vi "UHR-Fleezers Control (host) - Lorentz v4.vi"() -> ()   [LabVIEW 2014] (continued)
        n2223 = Multiply(x="Base N trap periods", y="Period scale factor") -> ()  [unwired: 1 out]
        n2224 = local read "Cal sets to save"() -> (w3460:u32)
        n2225 = To Unsigned Quad Integer(1:w3456) -> (0:w3446:u64)
        n2226 = for "vector 0 to N -1" {
          N: w3432 -> [_]
          tunnel: [w3481] -> w3452 mode=indexing
          i -> [w3481]
        }
        n2227 = Multiply "Ticks/DMA"(x=w3459, y=w3464) -> (x*y=w3463:u32)
        n2228 = Multiply "Scaled osc period (s)"(x=w3446, y=2.5e-08) -> (x*y=w3458:dbl)
        "Trap OSC Period (s)" <- w3458
        n2229 = Reciprocal(x=w3458) -> (1/x=→"A cal freq (Hz)":dbl)
        n2230 = Multiply(x=w3452, y=6.283185307179586) -> (x*y=w3467:dbl[])
        n2231 = Quotient & Remainder(x=w3463, y=w3446) -> (x-y*floor(x/y)=w3439:u64, floor(x/y)=→"N osc / DMA":u64)
        "DMA remainder" <- w3439
        n2232 = Multiply "Total trap ticks"(x=w3460, y=w3463) -> (x*y=w3447:u32)
        n2233 = Divide(x=w3467, y=w3432) -> (x/y=w3468:dbl[])
        n2234 = Sine(x=w3468) -> (sin(x)=w3469:dbl[])
        n2235 = Quotient & Remainder(x=w3447, y=100) -> (x-y*floor(x/y)=w3442:u32, floor(x/y)=w3462:u32)
        "Total save/100 remainder" <- w3442
        n2236 = Multiply "Single period osc vector"(x=w3469, y="Trap osc amp (MHz)") -> (x*y=w3445:dbl[])
        n2237 = Quotient & Remainder(x=w3462, y=w3446) -> (x-y*floor(x/y)=w3441:u64, floor(x/y)=→"N osc/ (total save/100)":u64)
        "(total save/100) /osc period remainder" <- w3441
        n2238 = Quotient & Remainder(x=w3447, y=w3446) -> (x-y*floor(x/y)=w3440:u64)  [unwired: 1 out]
        "N trap osc periods per save remainder" <- w3440
        n2239 = call "IR AOM freq to word - vec.vi"("Frequency In (double vec, MHz)"=w3445) -> ("Frequency Word Out"=w3444:dbl[])
        n2240 = To Quad Integer(1:w3444) -> (0:w3443:i64[])
        n2241 = disable-structure shown="Disabled" {
          disable-tunnel: w3451 -> [w3473 _]
          disable-tunnel: w3443 -> [w3471 _]
          frame Disabled {
            n2242 = xnode "Read/Write Control"("FPGA VI Reference In"=w3473) -> ("FPGA VI Reference Out"=w3472:T50)  [unwired: 3 in, 1 out]
            n2243 = flat-sequence {
              tunnel: w3471 -> [w3476]
              tunnel: w3472 -> [w3475]
              frame #0 {
                n2244 = for "Write data to fpga memory" {
                  tunnel: w3475 -> [w3478]
                  tunnel: w3476 -> [_] mode=indexing
                  (unwired) TRUE ("Ready Write")
                  n2245 = xnode "Read/Write Control"("FPGA VI Reference In"=w3478) -> ("FPGA VI Reference Out"=w3477:T50)  [unwired: 4 in, 1 out]
                  n2246 = while {
                    tunnel: w3477 -> [w3479]
                    stop <- _ continue-if-true
                    n2247 = xnode "Read/Write Control"("FPGA VI Reference In"=w3479) -> ()  [unwired: 1 in, 3 out]
                  }
                }
                "Writing waveform to fpga memory" <- TRUE ("Writing waveform to fpga memory")
              }
              frame #1 {
                n2248 = local write "Writing waveform to fpga memory"(FALSE ("Writing waveform to fpga memory")) -> ()
              }
            }
          }
          frame Enabled {
          }
        }
        n2249 = Equal?(x=w3441, y=w3438) -> (x = y?=w3436:bool)
        n2250 = Equal?(x=w3442, y=w3438) -> (x = y?=w3437:bool)
        n2251 = Equal?(x=w3439, y=w3438) -> (x = y?=w3434:bool)
        n2252 = Equal?(x=w3440, y=w3438) -> (x = y?=w3435:bool)
        n2253 = Compound Arithmetic op=AND(w3437, w3436, w3435, w3434) -> (→"Good freq?":bool)
      }
      event "Osc trap cont.", "Osc traps", "T1 Osc Enable", "T2 Osc Enable": Value Change {
        n2254 = event-data() -> ()  [unwired: 7 out]
        n2255 = disable-structure shown="Disabled" {
          disable-tunnel: w3482 -> [w3485 _]
          frame Disabled {
            n2256 = xnode "Read/Write Control"("FPGA VI Reference In"=w3485, "Trap 1 osc enable"="T1 Osc Enable", "Trap 2 osc enable"="T2 Osc Enable") -> ()  [unwired: 1 in, 2 out]
          }
          frame Enabled {
          }
        }
      }
      event "Pressure Pump Voltage (+/-10V)": Value Change {
        n2257 = event-data() -> ()  [unwired: 7 out]
        n2258 = disable-structure shown="Disabled" {
          disable-tunnel: w3486 -> [w3490 _]
          frame Disabled {
            n2259 = Divide(x="Pressure Pump Voltage (+/-10V)", y=10.0) -> (x/y=w3487:dbl)
            n2260 = Multiply(x=w3487, y=32767.0) -> (x*y=w3488:dbl)
            n2261 = xnode "Read/Write Control"("FPGA VI Reference In"=w3490, "Pressure Pump"=w3488) -> ()  [unwired: 1 in, 2 out]
          }
          frame Enabled {
          }
        }
      }
      event "Dynamic Force FB (ronen)": Value Change {
        # "Added by ronen - for feedback on trap position by changing the actual frequency and not the set frequency - for increasing the range of feedback."
        n2262 = event-data() -> ()  [unwired: 7 out]
        n2263 = xnode "Read/Write Control"("FPGA VI Reference In"=w3494, "Dynamic Force FB (Ronen)"="Dynamic Force FB (ronen)") -> ()  [unwired: 1 in, 2 out]
      }
      event "Read Setpoint Correction File": Value Change {
        n2264 = event-data() -> ()  [unwired: 7 out]
        n2265 = local write "Read Setpoint Correction File"(FALSE ("Read Setpoint Correction File")) -> ()
        n2266 = Open/Create/Replace File(file path (use dialog)="Setpoint Correction Offset File", operation (0:open)=T39."open", access (0:read/write)=enum16{"read/write", "read-only", "write-only"}."read-only") -> (refnum out=w3518:refnum<file>)  [unwired: 1 in, 4 out]
        n2267 = Deny Access(7:w3518) -> (3:w3517:refnum<file>)  [unwired: 1 in, 2 out]
        n2268 = Read from Binary File(5:0.0, 9:T38."big-endian, network order" ("byte order (0:big-endian, network order)"), 10:-1 ("count (1)"), 11:w3517) -> (2:w3511:dbl[], 3:w3516:refnum<file>)  [unwired: 1 in, 3 out]
        n2269 = Close File(refnum=w3516) -> ()  [unwired: 1 in, 2 out]
        n2270 = Array Subset(array=w3511, index=3) -> (w3512:dbl[])  [unwired: 1 in]
        n2271 = Index Array(array=w3511, index=0) -> (element=w3500:dbl)
        n2272 = local read "T2 calibration"() -> (w3499:T8)
        n2273 = local read "T1 calibration"() -> (w3507:T9)
        n2274 = local write "Offset file step size"(w3500) -> ()
        n2275 = Unbundle By Name(w3499) -> ("T2 alpha_x (nm/V)"=w3502:dbl, "T2 kappa_x (pN/nm)"=w3501:dbl)
        n2276 = Unbundle By Name(w3507) -> ("T1 alpha_x (nm/V)"=w3504:dbl, "T1 kappa_x (pN/nm)"=w3503:dbl)
        n2277 = Multiply(x=w3504, y=w3503) -> (x*y=w3505:dbl)
        n2278 = Multiply(x=w3502, y=w3501) -> (x*y=w3506:dbl)
        n2279 = Decimate 1D Array(w3512) -> (w3509:dbl[], w3508:dbl[])  [unwired: 1 out]
        n2280 = Divide(x=w3506, y=w3505) -> (x/y=w3496:dbl)
        n2281 = property on="B factor" class="DigNum (strict)"("Val(Sgnl)"=w3496) -> ()  [unwired: 2 in, 2 out]
        n2282 = Multiply(x=w3508, y=w3496) -> (x*y=w3510:dbl[])
        n2283 = Subtract(x=w3509, y=w3510) -> (x-y=w3495:dbl[])
        n2284 = local read "Offset Values"() -> (w3498:T20)
        n2285 = Bundle By Name(cluster=w3498, "Trap 1X offset"=w3509, "Trap 2X offset"=w3508) -> (w3497:T20)
        n2286 = local write "Offset Values"(w3497) -> ()
        n2287 = property on="Setpoint offset\ncorrection values" class="Arr (strict)"("Val(Sgnl)"=w3495) -> ()  [unwired: 2 in, 2 out]
      }
      event "B factor", "Setpoint offset\ncorrection values", "Target Force (pN)": Value Change {
        w3555 = 6.0  # clock mult.
        w3556 = 49152000.0  # TCXO frequ.
        n2288 = event-data() -> ()  [unwired: 7 out]
        n2289 = local read "B factor"() -> (w3557:dbl)
        n2290 = xnode "Read/Write Control"("FPGA VI Reference In"=w3558, "B factor"=w3557) -> ("BD1 Frequency Out 1"=w3548:u64)  [unwired: 1 in, 2 out]
        n2291 = To Double Precision Float(number=w3548) -> (double precision float=w3554:dbl)
        n2292 = local read "BD 1 Frequency 2 (MHz)"() -> (w3546:dbl)
        n2293 = Multiply(x=w3556, y=w3555) -> (x*y=w3553:dbl)
        n2294 = Multiply(x=w3554, y=w3553) -> (x*y=w3552:dbl)
        n2295 = Scale By Power Of 2(n=-48, x=w3552) -> (x*2^n=w3550:dbl)
        n2296 = Divide(x=w3550, y=1000000.0) -> (x/y=w3547:dbl)
        n2297 = Subtract(x=w3546, y=w3547) -> (x-y=w3534:dbl)
        n2298 = local read "Target Force (pN)"() -> (w3545:dbl)
        n2299 = local read "T1 calibration"() -> (w3543:T9)
        n2300 = local read "Offset file step size"() -> (w3533:dbl)
        n2301 = local read "Setpoint offset\ncorrection values"() -> (w3530:dbl[])
        n2302 = Unbundle By Name(w3543) -> ("T1 alpha_x (nm/V)"=w3542:dbl, "T1 kappa_x (pN/nm)"=w3541:dbl)
        n2303 = Multiply(x=w3545, y=2.0) -> (x*y=w3539:dbl)
        n2304 = Divide(x=w3534, y=w3533) -> (x/y=w3532:dbl)
        n2305 = local read "Negate Diff?"() -> (w3536:bool)
        n2306 = To Long Integer(number=w3532) -> (32bit integer=w3531:i32)
        n2307 = Multiply(x=w3542, y=w3541) -> (x*y=w3540:dbl)
        n2308 = Index Array(array=w3530, index=w3531) -> (element=w3528:dbl)
        n2309 = Divide(x=w3539, y=w3540) -> (x/y=w3535:dbl)
        n2310 = Select(t=1, s=w3536, f=-1) -> (s? t:f=w3529:i32)
        n2311 = Multiply(x=w3529, y=w3528) -> (x*y=w3527:dbl)
        n2312 = Add(x=w3535, y=w3527) -> (x+y=w3526:dbl)
        n2313 = To Fixed-Point(number=w3526) -> (fixed-point=w3525:fxp<+/-,16,1>)  [unwired: 1 in]
        n2314 = property on="Trap Pos FB SP" class="DigNum (strict)"("Val(Sgnl)"=w3525) -> ()  [unwired: 2 in, 2 out]
      }
      event "Trap 3 (ON/OFF)", "T3 Y (V)", "T3 X (V)": Value Change {
        n2315 = event-data() -> ()  [unwired: 7 out]
        n2316 = case shown="False" "Trap 3 (ON/OFF)" {
          tunnel: [5.0 0.0] -> w3560
          frame False {
          }
          frame True {
          }
        }
        n2317 = Multiply(x="T3 X (V)", y=32767.0) -> (x*y=w3576:dbl)
        n2318 = Multiply(x="T3 Y (V)", y=32767.0) -> (x*y=w3573:dbl)
        n2319 = Divide(x=w3576, y=10.0) -> (x/y=w3577:dbl)
        n2320 = Divide(x=w3573, y=10.0) -> (x/y=w3572:dbl)
        n2321 = To Unsigned Word Integer(number=w3577) -> (unsigned 16bit integer=w3566:u16)
        n2322 = To Unsigned Word Integer(number=w3572) -> (unsigned 16bit integer=w3567:u16)
        n2323 = Multiply(x=w3560, y=32767.0) -> (x*y=w3563:dbl)
        n2324 = Divide(x=w3563, y=10.0) -> (x/y=w3562:dbl)
        n2325 = To Unsigned Word Integer(number=w3562) -> (unsigned 16bit integer=w3559:u16)
        n2326 = xnode "Read/Write Control"("FPGA VI Reference In"=w3568, "Piezo Trap X (AO5)"=w3566, "Piezo Trap Y (AO4)"=w3567, "Piezo Trap ON/Off (AO3)"=w3559) -> ()  [unwired: 1 in, 2 out]
      }
      event "Cursor control.X", "Cursor control.Y": Value Change {
        # "If turning cursor control off, update the piezo controls"
        n2327 = event-data() -> ()  [unwired: 7 out]
        n2328 = xnode "Read/Write Control"("FPGA VI Reference In"=w3587) -> ("Piezo X out"=w3585:u16, "Piezo Y out"=w3581:u16)  [unwired: 1 in, 2 out]
        n2329 = local read "Cursor control"() -> (w3586:cluster{"X":bool, "Y":bool})
        n2330 = Unbundle By Name(w3586) -> ("X"=w3584:bool, "Y"=w3583:bool)
        n2331 = And(x=w3584, y=w3583) -> (x .and. y?=w3582:bool)
        n2332 = case shown="True" w3582 {
          tunnel: w3585 -> [w3592 _]
          tunnel: w3581 -> [w3590 _]
          frame False {
            w3589 = 3276.7
            n2333 = Divide(x=w3592, y=w3589) -> (x/y=w3591:dbl)
            n2334 = Divide(x=w3590, y=w3589) -> (x/y=w3588:dbl)
            n2335 = property on="T3 X (V)" class="DigNum (strict)"("Val(Sgnl)"=w3591) -> ()  [unwired: 2 in, 2 out]
            n2336 = property on="T3 Y (V)" class="DigNum (strict)"("Val(Sgnl)"=w3588) -> ()  [unwired: 2 in, 2 out]
          }
          frame True {
          }
        }
      }
    }
    "error out 2" <- w1973
    n2337 = node-c288() -> ()  [unwired: 2 out]
  }
  n2338 = node-c288() -> (w85:T35)  [unwired: 4 out]
  n2339 = timed-loop "Mouse control: trap position (AOM deflection), set confocal spot from image" {
    tunnel: [w3593] -> w90
    timing: w85 -> [_]
    timing-out: [_] -> w84
    tunnel: w42 -> [w3594]
    stop <- w3593 stop-if-true
    n2340 = node-c288() -> ()  [unwired: 2 out]
    n2341 = event shown="[0] \"Pane\": Mouse Down" {
      selector: _ -> [_ _ _ _]
      dyn-events: _ -> [_ _ _ _]
      timeout: _ -> [_ _ _ _]
      tunnel: w3594 -> [w3597 _ _ _]
      tunnel: [_ _ TRUE _] -> w3593
      event Mouse Down {
        n2342 = event-data() -> ("Time"=w3599:u32, "Coords"=w3598:T12, "Button"=w3600:u16)  [unwired: 6 out]
        n2343 = case shown="1" w3600 {
          tunnel: w3599 -> [_ _ w3706]
          tunnel: w3598 -> [_ w3637 w3704]
          tunnel: w3597 -> [_ _ w3700]
          frame 0, Default {
          }
          frame 1 {
            n2344 = property on="APD 2" class="ImageControl"() -> ("Displayed Image Position"=w3607:cluster{"Left":i32, "Top":i32})  [unwired: 2 in, 2 out]
            n2345 = property on="APD 1" class="ImageControl"() -> ("Displayed Image Position"=w3636:cluster{"Left":i32, "Top":i32})  [unwired: 2 in, 2 out]
            n2346 = property on="Detection Laser X" class="ImageControl"() -> ("Displayed Image Position"=w3633:cluster{"Left":i32, "Top":i32})  [unwired: 2 in, 2 out]
            n2347 = property on="Detection Laser Y" class="ImageControl"() -> ("Displayed Image Position"=w3632:cluster{"Left":i32, "Top":i32})  [unwired: 2 in, 2 out]
            n2348 = property on="APD 2" class="ImageControl"() -> ("Displayed Image Size"=w3606:cluster{"Width":u32, "Height":u32})  [unwired: 2 in, 2 out]
            n2349 = property on="APD 1" class="ImageControl"() -> ("Displayed Image Size"=w3634:cluster{"Width":u32, "Height":u32})  [unwired: 2 in, 2 out]
            n2350 = property on="Detection Laser X" class="ImageControl"() -> ("Displayed Image Size"=w3635:cluster{"Width":u32, "Height":u32})  [unwired: 2 in, 2 out]
            n2351 = property on="Detection Laser Y" class="ImageControl"() -> ("Displayed Image Size"=w3631:cluster{"Width":u32, "Height":u32})  [unwired: 2 in, 2 out]
            n2352 = Unbundle By Name(w3606) -> ("Width"=w3603:u32, "Height"=w3602:u32)
            n2353 = Unbundle By Name(w3607) -> ("Left"=w3605:i32, "Top"=w3604:i32)
            n2354 = Unbundle By Name(w3634) -> ("Width"=w3628:u32, "Height"=w3627:u32)
            n2355 = Unbundle By Name(w3635) -> ("Width"=w3624:u32, "Height"=w3623:u32)
            n2356 = Unbundle By Name(w3631) -> ("Width"=w3620:u32, "Height"=w3619:u32)
            n2357 = Unbundle By Name(w3636) -> ("Left"=w3630:i32, "Top"=w3629:i32)
            n2358 = Unbundle By Name(w3633) -> ("Left"=w3626:i32, "Top"=w3625:i32)
            n2359 = Unbundle By Name(w3632) -> ("Left"=w3622:i32, "Top"=w3621:i32)
            n2360 = Bundle("Left"=w3605, "Top"=w3604, "Width"=w3603, "Height"=w3602) -> (w3601:T58)  [unwired: 1 in]
            n2361 = Bundle("Left"=w3630, "Top"=w3629, "Width"=w3628, "Height"=w3627) -> (w3618:T58)  [unwired: 1 in]
            n2362 = Bundle("Left"=w3626, "Top"=w3625, "Width"=w3624, "Height"=w3623) -> (w3617:T58)  [unwired: 1 in]
            n2363 = Bundle("Left"=w3622, "Top"=w3621, "Width"=w3620, "Height"=w3619) -> (w3616:T58)  [unwired: 1 in]
            n2364 = Build Cluster Array(w3601, w3618, w3617, w3616) -> (w3615:T59)
            n2365 = for {
              tunnel: w3637 -> [w3648]
              tunnel: w3615 -> [w3649] mode=indexing
              shift-right: [w3646] -> w3613
              shift-left: TRUE -> [w3647]
              shift-right: [w3645] -> w3611
              shift-left: _ -> [w3641]
              shift-right: [w3644] -> w3610
              shift-left: _ -> [w3640]
              shift-right: [w3643] -> w3609
              shift-left: _ -> [w3639]
              shift-right: [w3642] -> w3608
              shift-left: _ -> [w3638]
              n2366 = case shown="True" w3647 {
                selector: w3647 -> [w3654 _]
                tunnel: w3649 -> [_ w3663]
                tunnel: w3648 -> [_ w3661]
                tunnel: [w3654 w3659] -> w3646
                tunnel: [w3653 w3658] -> w3645
                tunnel: [w3652 w3657] -> w3644
                tunnel: [w3651 w3656] -> w3643
                tunnel: [w3650 w3655] -> w3642
                tunnel: w3641 -> [w3653 _]
                tunnel: w3640 -> [w3652 _]
                tunnel: w3639 -> [w3651 _]
                tunnel: w3638 -> [w3650 _]
                frame False {
                }
                frame True {
                  n2367 = Unbundle(w3663) -> (w3662:T58)
                  n2368 = call "isclickinwindow.vi"("Image Param"=w3662, "Point32"=w3661) -> ("4 Y"=w3655:i32, "3 Height"=w3656:i32, "2 X"=w3657:i32, "1 Width"=w3658:i32, "In image?"=w3660:bool)  [unwired: 1 in]
                  n2369 = Not(x=w3660) -> (.not. x?=w3659:bool)
                }
              }
            }
            n2370 = Not(x=w3613) -> (.not. x?=w3612:bool)
            n2371 = case shown="True" w3612 {
              tunnel: w3610 -> [_ w3677]
              tunnel: w3608 -> [_ w3676]
              tunnel: w3611 -> [_ w3675]
              tunnel: w3609 -> [_ w3674]
              frame False {
              }
              frame True {
                w3664 = FALSE ("Get Point")
                n2372 = local read "Scan lines (y)"() -> (w3679:u64)
                n2373 = disable-structure shown="Disabled" {
                  frame Disabled {
                  }
                  frame Enabled {
                  }
                }
                n2374 = local read "Actual MCL Inc (V)"() -> (w3673:dbl)
                n2375 = local read "Scan steps (MCL)"() -> (w3678:u64)
                n2376 = Divide "Y Pix/step"(x=w3674, y=w3679) -> (x/y=w3686:dbl)
                n2377 = Divide "Y V/pix"(x=w3673, y=w3686) -> (x/y=w3685:dbl)
                n2378 = Divide "Y half step offset"(x=w3673, y=2.0) -> (x/y=w3687:dbl)
                n2379 = Divide "X pix/step"(x=w3675, y=w3678) -> (x/y=w3684:dbl)
                n2380 = Negate(x=w3687) -> (-x=w3688:dbl)
                n2381 = local read "Initial Y"() -> (w3694:dbl)
                n2382 = Multiply(x=w3676, y=w3685) -> (x*y=w3695:dbl)
                n2383 = Divide "X half step offset"(x=w3673, y=2.0) -> (x/y=w3681:dbl)
                n2384 = Divide "X V/pix"(x=w3673, y=w3684) -> (x/y=w3683:dbl)
                n2385 = Multiply(x=w3673, y=w3678) -> (x*y=w3690:dbl)
                n2386 = Compound Arithmetic op=ADD(w3688, w3695, w3694) -> (w3665:dbl)
                "Pointer Y (V)" <- w3665
                n2387 = Multiply(x=w3683, y=w3677) -> (x*y=w3692:dbl)
                n2388 = Negate(x=w3681) -> (-x=w3680:dbl)
                n2389 = local read "Initial X"() -> (w3693:dbl)
                n2390 = Negate(x=w3692) -> (-x=w3691:dbl)
                n2391 = Compound Arithmetic op=ADD(w3680, w3690, w3693, w3691) -> (w3666:dbl)
                "Pointer X (V)" <- w3666
                n2392 = case shown="True" "Set High F Confocal Spot (X-Y)" {
                  tunnel: w3666 -> [_ w3696]
                  tunnel: w3665 -> [_ w3697]
                  frame False {
                  }
                  frame True {
                    "Confocal Y 2 (V)" <- w3697
                    "Confocal X 2 (V)" <- w3696
                  }
                }
                n2393 = Or(x="Set X Only", y="Set Confocal Spot (X-Y)") -> (x .or. y?=w3669:bool)
                n2394 = Or(x="Set Confocal Spot (X-Y)", y="Set Y Only") -> (x .or. y?=w3668:bool)
                n2395 = case shown="True" w3669 {
                  tunnel: w3666 -> [_ w3698]
                  frame False {
                  }
                  frame True {
                    n2396 = property on="AO2" class="Slide (strict)"("Val(Sgnl)"=w3698) -> ()  [unwired: 2 in, 2 out]
                    "Confocal X 1 (V)" <- w3698
                  }
                }
                n2397 = case shown="True" w3668 {
                  tunnel: w3665 -> [_ w3699]
                  frame False {
                  }
                  frame True {
                    n2398 = property on="AO1" class="Slide (strict)"("Val(Sgnl)"=w3699) -> ()  [unwired: 2 in, 2 out]
                    "Confocal Y 1 (V)" <- w3699
                  }
                }
                n2399 = local write "Set High F Confocal Spot (X-Y)"(w3664) -> ()
                n2400 = local write "Set Confocal Spot (X-Y)"(w3664) -> ()
                n2401 = local write "Set X Only"(w3664) -> ()
                n2402 = local write "Set Y Only"(w3664) -> ()
              }
            }
          }
          frame 3 {
            n2403 = local read "BD 2 Frequency 1 (MHz)"() -> (w3701:dbl)
            n2404 = local read "BD 1 Frequency 1 (MHz)"() -> (w3702:dbl)
            n2405 = local write "Manipulating Trap"(TRUE ("Manipulating Trap")) -> ()
            n2406 = local write "Coords"(T12 {"Horizontal"=0, "Vertical"=0} ("Coords")) -> ()
            n2407 = while {
              tunnel: w3706 -> [w3711]
              tunnel: w3704 -> [w3710]
              tunnel: w3702 -> [w3709]
              tunnel: w3701 -> [w3708]
              tunnel: w3700 -> [w3707]
              stop <- w3712 stop-if-true
              n2408 = event shown="[0] \"Pane\": Mouse Move" {
                selector: _ -> [_ _]
                dyn-events: _ -> [_ _]
                timeout: _ -> [_ _]
                tunnel: ["Force Manip Abort" w3776] -> w3712
                tunnel: w3711 -> [w3719 _]
                tunnel: w3710 -> [w3717 _]
                tunnel: w3709 -> [w3716 _]
                tunnel: w3708 -> [w3715 _]
                tunnel: w3707 -> [w3713 _]
                event Mouse Move {
                  n2409 = event-data() -> ("Time"=w3720:u32, "Coords"=w3721:T12)  [unwired: 3 out]
                  n2410 = Less?(x=w3720, y=w3719) -> (x < y?=w3718:bool)
                  n2411 = case "Makes sure old motion events prior to mouse click aren't used" shown="False" w3718 {
                    tunnel: w3721 -> [w3763 _]
                    tunnel: w3717 -> [w3764 _]
                    tunnel: w3716 -> [w3738 _]
                    tunnel: w3715 -> [w3737 _]
                    tunnel: w3713 -> [w3722 _]
                    frame False {
                      n2412 = Subtract(x=w3763, y=w3764) -> (x-y=w3762:T12)
                      "Coords" <- w3762
                      n2413 = local read "Y RF Frequency Limits (MHz)"() -> (w3723:T24)
                      n2414 = To Double Precision Float(number=w3762) -> (double precision float=w3761:cluster{"Horizontal":dbl, "Vertical":dbl})
                      n2415 = Multiply(x=cluster{"Horizontal":dbl, "Vertical":dbl} {"Horizontal"=-1.0, "Vertical"=1.0}, y="Manipulation Scaling") -> (x*y=w3757:cluster{"Horizontal":dbl, "Vertical":dbl})
                      n2416 = local read "X RF Frequency Limits (MHz)"() -> (w3724:T24)
                      n2417 = Multiply(x=w3761, y=w3757) -> (x*y=w3759:cluster{"Horizontal":dbl, "Vertical":dbl})
                      n2418 = Unbundle By Name(w3759) -> ("Horizontal"=w3754:dbl, "Vertical"=w3758:dbl)
                      n2419 = Unbundle By Name(w3723) -> ("Maximum"=w3726:dbl, "Minimum"=w3725:dbl)
                      n2420 = Boolean To (0,1)(Boolean="Manip. X?") -> (0, 1=w3752:i16)
                      n2421 = Boolean To (0,1)(Boolean="Manip. Y?") -> (0, 1=w3749:i16)
                      n2422 = local read "BD 1 Frequency 2 (MHz)"() -> (w3740:dbl)
                      n2423 = Multiply(x=w3758, y=w3749) -> (x*y=w3751:dbl)
                      n2424 = Multiply(x=w3752, y=w3754) -> (x*y=w3755:dbl)
                      n2425 = local read "BD 2 Frequency 2 (MHz)"() -> (w3739:dbl)
                      n2426 = Unbundle By Name(w3724) -> ("Maximum"=w3728:dbl, "Minimum"=w3727:dbl)
                      n2427 = Add(x=w3737, y=w3751) -> (x+y=w3730:dbl)
                      n2428 = Add(x=w3738, y=w3755) -> (x+y=w3732:dbl)
                      n2429 = In Range and Coerce(upper limit=w3728, x=w3732, lower limit=w3727) -> (coerced(x)=w3731:dbl)  [unwired: 1 out]
                      n2430 = In Range and Coerce(upper limit=w3726, x=w3730, lower limit=w3725) -> (coerced(x)=w3729:dbl)  [unwired: 1 out]
                      n2431 = Subtract(x=w3731, y=w3740) -> (x-y=w3748:dbl)
                      n2432 = Subtract(x=w3729, y=w3739) -> (x-y=w3747:dbl)
                      n2433 = Square(x=w3748) -> (x^2=w3746:dbl)
                      n2434 = Square(x=w3747) -> (x^2=w3745:dbl)
                      n2435 = Add(x=w3746, y=w3745) -> (x+y=w3744:dbl)
                      n2436 = Square Root(x=w3744) -> (sqrt(x)=w3741:dbl)
                      n2437 = In Range and Coerce(upper limit="Limit Max (MHz)", x=w3741, lower limit="Limit Min (MHz)") -> (In Range?=w3734:bool)  [unwired: 1 out]
                      n2438 = Not(x="Limits Enable") -> (.not. x?=w3733:bool)
                      n2439 = Or(x=w3734, y=w3733) -> (x .or. y?=w3735:bool)
                      n2440 = case shown="True" w3735 {
                        tunnel: w3741 -> [_ w3766]
                        tunnel: w3731 -> [_ w3773]
                        tunnel: w3740 -> [_ w3772]
                        tunnel: w3729 -> [_ w3771]
                        tunnel: w3739 -> [_ w3770]
                        tunnel: w3724 -> [_ w3768]
                        tunnel: w3723 -> [_ w3767]
                        tunnel: w3722 -> [_ w3765]
                        frame False {
                        }
                        frame True {
                          n2441 = local read "BD 1 Frequency 3 (MHz)"() -> (w3774:dbl)
                          n2442 = local read "BD 2 Frequency 3 (MHz)"() -> (w3769:dbl)
                          n2443 = local write "Trap Delta (MHz)"(w3766) -> ()
                          n2444 = call "set RF board frequency - interlace.vi"("Board 2 Frequency Limits"=w3767, "Board 1 Frequency Limits"=w3768, "FPGA VI Reference In"=w3765, "Board 2 Frequency 3 (MHz)"=w3769, "Board 1 Frequency 3 (MHz)"=w3774, "Board 2 Frequency 2 (MHz)"=w3770, "Board 2 Frequency 1 (MHz)"=w3771, "Board 1 Frequency 2 (MHz)"=w3772, "Board 1 Frequency 1  (MHz)"=w3773) -> ()  [unwired: 1 in, 2 out]
                          n2445 = local write "BD 2 Frequency 1 (MHz)"(w3771) -> ()
                          n2446 = local write "BD 1 Frequency 1 (MHz)"(w3773) -> ()
                        }
                      }
                    }
                    frame True {
                    }
                  }
                }
                event Mouse Up {
                  n2447 = event-data() -> ("Button"=w3775:u16)  [unwired: 8 out]
                  n2448 = case shown="3" w3775 {
                    tunnel: [FALSE TRUE] -> w3776
                    frame 0, Default {
                    }
                    frame 3 {
                      n2449 = local read "Trap Delta (MHz)"() -> (w3778:dbl)
                      n2450 = property on="Initial delta (MHz)" class="DigNum (strict)"("Val(Sgnl)"=w3778) -> ()  [unwired: 2 in, 2 out]
                      n2451 = local write "Manipulating Trap"(FALSE ("Manipulating Trap")) -> ()
                    }
                  }
                }
              }
            }
          }
        }
      }
      event Timeout {
        n2452 = event-data() -> ()  [unwired: 4 out]
      }
      event "Stop All": Mouse Down {
        n2453 = event-data() -> ()  [unwired: 9 out]
      }
      event Mouse Move {
        n2454 = event-data() -> ()  [unwired: 6 out]
      }
    }
    n2455 = node-c288() -> ()  [unwired: 2 out]
  }
  n2456 = node-c288(3 ("Processor")) -> (w81:T35)  [unwired: 3 out]
  n2457 = node-c288(i64 1 ("Period"), 1 ("Processor")) -> (w89:T35)  [unwired: 2 in, 2 out]
  n2458 = timed-loop "Oscillate Trap/AOM (fishing, conjugate plane alignment)" {
    tunnel: [w3784] -> w86
    timing: w81 -> [_]
    timing-out: [_] -> w80
    tunnel: w42 -> [w3783]
    tunnel: w30 -> [w3782]
    stop <- w3784 stop-if-true
    n2459 = node-c288() -> ()  [unwired: 2 out]
    n2460 = event shown="[2] \"Start assembly line\": Value Change" {
      selector: _ -> [_ _ _ _]
      dyn-events: _ -> [_ _ _ _]
      timeout: _ -> [_ _ _ _]
      tunnel: [FALSE ("Stop All") _ _ w4457] -> w3784
      tunnel: w3783 -> [w3787 _ _ _]
      tunnel: w3782 -> [_ _ w4392 _]
      event "Oscillate Set 1", "Fish for Tether": Value Change {
        n2461 = event-data() -> ()  [unwired: 6 out]
        n2462 = local read "Oscillate Set 1"() -> (w3791:bool)
        n2463 = Or(x=w3791, y="Fish for Tether") -> (x .or. y?=w3789:bool)
        n2464 = case shown="True" w3789 {
          tunnel: "Fish for Tether" -> [_ w3794]
          tunnel: w3787 -> [_ w3792]
          frame False {
          }
          frame True {
            n2465 = case shown="True" w3794 {
              selector: w3794 -> [w3797 w3803]
              tunnel: [w3797 w3803] -> w3793
              frame False {
              }
              frame True {
                n2466 = local write "Scan axis 2"(TRUE) -> ()
                n2467 = local write "Tether"(FALSE ("Tether")) -> ()
                n2468 = local read "Flow ON during cal?"() -> (w3798:bool)
                n2469 = property on="Trap Delta (MHz)" class="DigNum (strict)"("Val(Sgnl)"="Furthest Delta (MHz)") -> ()  [unwired: 2 in, 2 out]
                n2470 = Or(x="Flow ON during \nfishing?", y=w3798) -> (x .or. y?=w3799:bool)
                n2471 = Wait (ms)(milliseconds to wait=u32 500) -> ()  [unwired: 1 out]
                n2472 = property on="Sample Channel\nFlow" class="Bool (strict)"("Val(Sgnl)"=w3799) -> ()  [unwired: 2 in, 2 out]
              }
            }
            n2473 = node-c288() -> (w3796:T35)  [unwired: 1 in, 3 out]
            n2474 = timed-loop "Oscillate AOD" {
              timing: w3796 -> [_]
              timing-out: [_] -> w3795
              tunnel: w3793 -> [w3807]
              tunnel: w3792 -> [w3806]
              i -> [w3815]
              stop <- w3813 stop-if-true
              n2475 = node-c288() -> (w3814:i64)  [unwired: 1 out]
              n2476 = flat-sequence {
                tunnel: w3815 -> [w3842]
                tunnel: w3814 -> [w3841]
                tunnel: w3807 -> [w3825]
                tunnel: [w3825] -> w3812
                tunnel: [w3824] -> w3811
                tunnel: [w3823] -> w3810
                tunnel: [w3820] -> w3808
                tunnel: w3806 -> [w3816]
                tunnel: w3812 -> [w3889]
                tunnel: w3811 -> [w3887]
                tunnel: w3810 -> [w3886]
                tunnel: [w3885] -> w3809
                tunnel: w3808 -> [w3884]
                tunnel: [w3961] -> w3813
                tunnel: w3809 -> [w3960]
                frame #0 {
                  # "w (rad/s)"
                  # "t (s)"
                  n2477 = Divide(x=w3841, y=i64 1000) -> (x/y=w3817:dbl)
                  n2478 = local read "BD 1 Frequency 2 (MHz)"() -> (w3819:dbl)
                  n2479 = Multiply(x="Osc. freq. (Hz)", y=6.283185307179586) -> (x*y=w3839:dbl)
                  n2480 = Multiply(x=w3817, y=w3842) -> (x*y=w3838:dbl)
                  n2481 = Multiply(x=w3839, y=w3838) -> (x*y=w3822:dbl)
                  n2482 = local read "BD 1 Frequency 1 (MHz)"() -> (w3827:dbl)
                  n2483 = case shown="True" w3825 {
                    tunnel: w3822 -> [w3848 w3867]
                    tunnel: w3827 -> [_ w3875]
                    tunnel: w3819 -> [_ w3876]
                    tunnel: [w3845 w3871] -> w3818
                    tunnel: [FALSE w3849] -> w3823
                    tunnel: [0.0 w3863] -> w3820
                    frame False {
                      n2484 = Sine(x=w3848) -> (sin(x)=w3846:dbl)
                      n2485 = Multiply(x=w3846, y="Osc. amp. (MHz)") -> (x*y=w3845:dbl)
                    }
                    frame True {
                      # "trap position goes from 0 to 1 (0 is when it is furthest away, 1 is when closest)\nso we want to test for tether only when farther away, or x < 1"
                      # "quit if taking too long"
                      # "oscillate the trap"
                      # "Test for tether"
                      n2486 = local read "Vec Mean of T1 T2"() -> (w3852:dbl[])
                      "Trigger Signal" <- w3852
                      n2487 = Cosine(x=w3867) -> (cos(x)=w3879:dbl)
                      n2488 = Subtract(x=w3876, y=w3875) -> (x-y=w3874:dbl)
                      n2489 = Decrement(x=w3879) -> (x-1=w3878:dbl)
                      n2490 = Subtract(x=w3874, y="Closest Delta (MHz)") -> (x-y=w3872:dbl)
                      n2491 = Divide(x=w3878, y=-2.0) -> (x/y=w3862:dbl)
                      n2492 = Greater?(x=w3852, y="Stop F (pN)") -> (0:w3869:bool[])
                      n2493 = Multiply(x=w3862, y=w3872) -> (x*y=w3871:dbl)
                      n2494 = Less?(x=w3862, y="Fish mask thresh") -> (x < y?=w3861:bool)
                      n2495 = Boolean To (0,1)(Boolean=w3861) -> (0, 1=w3859:i16)
                      n2496 = Multiply(x=w3859, y=w3852) -> (x*y=w3858:dbl[])
                      n2497 = Divide(x=w3867, y=6.283185307179586) -> (x/y=w3866:dbl)
                      n2498 = Round Toward +Infinity(x=w3866) -> (ceil(x): smallest int >= x=w3863:dbl)
                      "Attempts" <- w3863
                      n2499 = Greater?(x=w3858, y="Stop F (pN) (mask)") -> (0:w3856:bool[])
                      n2500 = Or Array Elements(Boolean array=w3869) -> (logical OR=w3854:bool)
                      n2501 = Or Array Elements(Boolean array=w3856) -> (logical OR=w3853:bool)
                      n2502 = Greater?(x=w3863, y="Attempt Limit") -> (0:w3865:bool)
                      n2503 = case shown="True" w3865 {
                        frame False {
                        }
                        frame True {
                          n2504 = local write "Fish for Tether"(FALSE ("Fish for Tether")) -> ()
                          n2505 = call <vilib>:"Beep.vi"() -> ()  [unwired: 3 in, 9 out]
                          n2506 = local read "Messages"() -> (w3881:string)
                          n2507 = call "Update messages.vi"("Message to add"="Tether fishing timeout." ("Messages"), "Old message string"=w3881) -> ("New message string"=→"Messages":string)
                        }
                      }
                      n2508 = Select(t=w3854, s="Normal (on) or masked test (off)", f=w3853) -> (s? t:f=w3851:bool)
                      n2509 = And(x="Stop Fishing When Tether", y=w3851) -> (x .and. y?=w3849:bool)
                    }
                  }
                  n2510 = local read "BD 2 Frequency 1 (MHz)"() -> (w3826:dbl)
                  n2511 = Select(t=w3827, s="Scan axis 2", f=w3826) -> (s? t:f=w3830:dbl)
                  n2512 = Add(x=w3818, y=w3830) -> (x+y=w3824:dbl)
                  n2513 = Select(t=w3824, s="Scan axis 2", f=w3827) -> (s? t:f=w3833:dbl)
                  n2514 = Select(t=w3826, s="Scan axis 2", f=w3824) -> (s? t:f=w3832:dbl)
                  n2515 = local read "BD 2 Frequency 2 (MHz)"() -> (w3835:dbl)
                  n2516 = local read "BD 2 Frequency 3 (MHz)"() -> (w3834:dbl)
                  n2517 = local read "Y RF Frequency Limits (MHz)"() -> (w3828:T24)
                  n2518 = local read "X RF Frequency Limits (MHz)"() -> (w3829:T24)
                  n2519 = local read "BD 1 Frequency 3 (MHz)"() -> (w3836:dbl)
                  n2520 = call "set RF board frequency - interlace.vi"("Board 2 Frequency Limits"=w3828, "Board 1 Frequency Limits"=w3829, "FPGA VI Reference In"=w3816, "Board 2 Frequency 3 (MHz)"=w3834, "Board 1 Frequency 3 (MHz)"=w3836, "Board 2 Frequency 2 (MHz)"=w3835, "Board 2 Frequency 1 (MHz)"=w3832, "Board 1 Frequency 2 (MHz)"=w3819, "Board 1 Frequency 1  (MHz)"=w3833) -> ()  [unwired: 1 in, 2 out]
                }
                frame #1 {
                  n2521 = And(x=w3889, y=w3886) -> (x .and. y?=w3888:bool)
                  n2522 = case "Only if were fishing and now formed tether" shown="True" w3888 {
                    tunnel: w3887 -> [w3891 w3906]
                    tunnel: [w3890 w3905] -> w3885
                    tunnel: w3884 -> [_ w3901]
                    frame False {
                      n2523 = local read "Fish for Tether"() -> (w3890:bool)
                      n2524 = case shown="False" w3890 {
                        tunnel: w3891 -> [w3892 _]
                        frame False {
                          n2525 = property on="BD 1 Frequency 1 (MHz)" class="DigNum (strict)"("Val(Sgnl)"=w3892) -> ()  [unwired: 2 in, 2 out]
                        }
                        frame True {
                        }
                      }
                    }
                    frame True {
                      w3905 = FALSE ("Fish for Tether")
                      n2526 = call <vilib>:"Beep.vi"() -> ()  [unwired: 3 in, 9 out]
                      n2527 = Number To Decimal String(number=w3901, width (-)=i16 1) -> (decimal integer string=w3899:string)
                      n2528 = Concatenate Strings("Formed tether in ", w3899, " attempt(s)." ("string")) -> (w3896:string)
                      n2529 = local read "Messages"() -> (w3903:string)
                      n2530 = local write "Fish for Tether"(w3905) -> ()
                      n2531 = call "Update messages.vi"("Message to add"=w3896, "Old message string"=w3903) -> ("New message string"=w3902:string)
                      n2532 = local write "Messages"(w3902) -> ()
                      n2533 = Get Date/Time In Seconds() -> (seconds since 1Jan1904=→"Time tether formed":timestamp)
                      n2534 = local read "Flow ON during cal?"() -> (w3893:bool)
                      n2535 = property on="Sample Channel\nFlow" class="Bool (strict)"("Val(Sgnl)"=w3893) -> (error out=w3894:errorcluster)  [unwired: 2 in, 1 out]
                      n2536 = case shown="\"2\", \"3\", \"4\", \"5\", \"6\"" "Then..." {
                        selector: "Then..." -> [_ w3909]
                        tunnel: w3906 -> [w3908 _]
                        tunnel: w3894 -> [_ _]
                        frame "1", Default {
                          n2537 = property on="BD 1 Frequency 1 (MHz)" class="DigNum (strict)"("Val(Sgnl)"=w3908) -> ()  [unwired: 2 in, 2 out]
                        }
                        frame "2", "3", "4", "5", "6" {
                          n2538 = flat-sequence {
                            tunnel: w3909 -> [w3911]
                            frame #0 {
                              n2539 = property on="Trap Delta (MHz)" class="DigNum (strict)"("Val(Sgnl)"="Move to Delta 1 (MHz)") -> ()  [unwired: 2 in, 2 out]
                            }
                            frame #1 {
                              n2540 = case shown="\"5\", \"6\"" w3911 {
                                selector: w3911 -> [w3914 w3924 _]
                                frame "3", "4" {
                                n2541 = flat-sequence {
                                tunnel: w3914 -> [w3915]
                                tunnel: [w3915] -> w3912
                                tunnel: [w3917] -> w3913
                                tunnel: w3912 -> [w3917]
                                tunnel: w3913 -> [w3921]
                                frame #0 {
                                n2542 = property on="Green Laser ON" class="Bool (strict)"("Val(Sgnl)"=TRUE ("Value (Signaling)")) -> ()  [unwired: 2 in, 2 out]
                                }
                                frame #1 {
                                n2543 = Multiply(x="Wait Before Save (s)", y=u32 1000 ("x")) -> (x*y=w3919:u32)
                                n2544 = Wait (ms)(milliseconds to wait=w3919) -> ()  [unwired: 1 out]
                                }
                                frame #2 {
                                n2545 = property on="Start Saving" class="Bool (strict)"("Value"=TRUE ("Start Saving")) -> ()  [unwired: 2 in, 2 out]
                                n2546 = case shown="\"4\"" w3921 {
                                frame Default {
                                }
                                frame "4" {
                                n2547 = property on="Fl. Triggered..." class="Bool (strict)"("Val(Sgnl)"=TRUE ("Value (Signaling)")) -> ()  [unwired: 2 in, 2 out]
                                }
                                }
                                }
                                }
                                }
                                frame "5", "6" {
                                n2548 = stacked-sequence {
                                tunnel: w3924 -> [_ _ _ _ _ _ w3936]
                                frame #0 {
                                n2549 = Replace Array Subset(array=u32[] [0] ("Index Values"), new element="Raster Set Upon Tether", index=0) -> (w3925:u32[])
                                n2550 = property on="Saved AOD Raster Scan Parameter Sets" class="Arr (strict)"("Index Values"=w3925) -> ()  [unwired: 2 in, 2 out]
                                }
                                frame #1 {
                                n2551 = Wait (ms)(milliseconds to wait=u32 500) -> ()  [unwired: 1 out]
                                }
                                frame #2 {
                                n2552 = property on="Load parameters" class="Bool (strict)"("Val(Sgnl)"=TRUE ("Value (Signaling)")) -> ()  [unwired: 2 in, 2 out]
                                n2553 = case shown="True" "Green ON During Raster" {
                                frame False {
                                }
                                frame True {
                                n2554 = property on="Green Laser ON" class="Bool (strict)"("Val(Sgnl)"=TRUE ("Value (Signaling)")) -> ()  [unwired: 2 in, 2 out]
                                }
                                }
                                }
                                frame #3 {
                                n2555 = Wait (ms)(milliseconds to wait=u32 500) -> ()  [unwired: 1 out]
                                }
                                frame #4 {
                                n2556 = property on="Trap Raster Scan" class="Bool (strict)"("Val(Sgnl)"=TRUE ("Value (Signaling)")) -> ()  [unwired: 2 in, 2 out]
                                }
                                frame #5 {
                                n2557 = Wait (ms)(milliseconds to wait=u32 2000) -> ()  [unwired: 1 out]
                                }
                                frame #6 {
                                n2558 = flat-sequence {
                                tunnel: w3936 -> [w3943]
                                frame #0 {
                                n2559 = while {
                                stop <- w3939 stop-if-true
                                n2560 = local read "Raster Scanning..."() -> (w3938:bool)
                                n2561 = local read "Saving..."() -> (w3941:bool)
                                n2562 = Wait (ms)(milliseconds to wait=u32 100) -> ()  [unwired: 1 out]
                                n2563 = Not(x=w3941) -> (.not. x?=w3940:bool)
                                n2564 = Not(x=w3938) -> (.not. x?=w3937:bool)
                                n2565 = And(x=w3940, y=w3937) -> (x .and. y?=w3939:bool)
                                }
                                }
                                frame #1 {
                                n2566 = local read "Tether"() -> (w3944:bool)
                                n2567 = case shown="True" w3944 {
                                tunnel: w3943 -> [_ w3946]
                                frame False {
                                n2568 = property on="Fish for Tether" class="Bool (strict)"("Val(Sgnl)"="Fish again after \nraster break?") -> ()  [unwired: 2 in, 2 out]
                                }
                                frame True {
                                n2569 = stacked-sequence {
                                tunnel: w3946 -> [_ w3950 _ _]
                                frame #0 {
                                n2570 = property on="Trap Delta (MHz)" class="DigNum (strict)"("Val(Sgnl)"="Move to Delta 2 (MHz)") -> ()  [unwired: 2 in, 2 out]
                                n2571 = case shown="True" "Flow ON after\ntether testing?" {
                                frame False {
                                }
                                frame True {
                                n2572 = property on="Sample Channel\nFlow" class="Bool (strict)"("Val(Sgnl)"=TRUE ("Value (Signaling)")) -> ()  [unwired: 2 in, 2 out]
                                }
                                }
                                }
                                frame #1 {
                                n2573 = flat-sequence {
                                tunnel: w3950 -> [w3952]
                                frame #0 {
                                n2574 = Wait (ms)(milliseconds to wait=u32 500) -> ()  [unwired: 1 out]
                                }
                                frame #1 {
                                n2575 = case shown="\"6\"" w3952 {
                                frame Default {
                                }
                                frame "6" {
                                n2576 = property on="Green Laser ON" class="Bool (strict)"("Val(Sgnl)"=TRUE ("Green Laser ON/Interlacing")) -> ()  [unwired: 2 in, 2 out]
                                }
                                }
                                }
                                frame #2 {
                                n2577 = Wait (ms)(milliseconds to wait=u32 500) -> ()  [unwired: 1 out]
                                }
                                frame #3 {
                                n2578 = local write "Start Saving"("Save at end (5, 6)") -> ()
                                }
                                }
                                }
                                frame #2 {
                                n2579 = local read "Bead Sep. Int. Time (s)"() -> (w3958:dbl)
                                n2580 = Multiply(x=w3958, y=1000.0) -> (x*y=w3957:dbl)
                                n2581 = Wait (ms)(milliseconds to wait=w3957) -> ()  [unwired: 1 out]
                                }
                                frame #3 {
                                n2582 = property on="Remove Offset" class="Bool (strict)"("Val(Sgnl)"=TRUE ("Value (Signaling)")) -> ()  [unwired: 2 in, 2 out]
                                }
                                }
                                }
                                }
                                }
                                }
                                }
                                }
                                }
                                frame "2", Default {
                                }
                              }
                            }
                          }
                        }
                      }
                      "Tether" <- "Tether Alarm?"
                    }
                  }
                }
                frame #2 {
                  n2583 = local read "Oscillate Set 1"() -> (w3965:bool)
                  n2584 = local read "Stop All"() -> (w3963:bool)
                  n2585 = Or(x=w3965, y=w3960) -> (x .or. y?=w3962:bool)
                  n2586 = Not(x=w3962) -> (.not. x?=w3964:bool)
                  n2587 = Compound Arithmetic op=OR(w3963, w3964) -> (w3961:bool)
                }
              }
              n2588 = node-c288() -> ()  [unwired: 2 out]
            }
            n2589 = node-c288(w3795) -> ()  [unwired: 1 out]
          }
        }
      }
      event "Fl. Triggered...": Value Change {
        n2590 = event-data() -> ()  [unwired: 7 out]
        n2591 = case shown="True" "Fl. Triggered..." {
          frame False {
          }
          frame True {
            n2592 = node-c288() -> (w3976:T35)  [unwired: 4 out]
            n2593 = timed-loop {
              timing: w3976 -> [_]
              timing-out: [_] -> w3975
              tunnel: "Action" -> [w3984]
              shift-right: [w3981] -> _
              shift-left: u8 255 -> [w3983]
              shift-right: [w3978] -> _
              shift-left: 255 -> [w3980]
              stop <- w3977 stop-if-true
              # "Reset confocal spot"
              n2594 = node-c288() -> ()  [unwired: 2 out]
              n2595 = flat-sequence {
                tunnel: w3984 -> [w4004]
                tunnel: w3983 -> [w4003]
                tunnel: [w4002] -> w3982
                tunnel: w3980 -> [w3989]
                tunnel: [w3988] -> w3979
                tunnel: [w4383] -> w3977
                tunnel: w3982 -> [w4382]
                tunnel: [w4382] -> w3981
                tunnel: [w4381] -> w3978
                tunnel: w3979 -> [w4381]
                frame #0 {
                  n2596 = local read "Delta Fl. 2"() -> (w4001:dbl)
                  n2597 = local read "Delta Fl. 1"() -> (w3996:dbl)
                  n2598 = Multiply(x="Fl. Delta Thresh. (kHz)", y=1000.0) -> (x*y=w3991:dbl)
                  n2599 = Select(t=w3996, s="APD to Watch", f=w4001) -> (s? t:f=w3992:dbl)
                  n2600 = Greater?(x=w3992, y=w3991) -> (0:w3997:bool)
                  n2601 = Or(x="Force Yank", y=w3997) -> (x .or. y?=w3995:bool)
                  n2602 = And(x=w3995, y="Yank when?") -> (x .and. y?=w3993:bool)
                  n2603 = case shown="True" w3993 {
                    tunnel: w4004 -> [w4007 w4208]
                    tunnel: w4003 -> [w4009 w4204]
                    tunnel: [w4009 w4202] -> w4002
                    tunnel: w3992 -> [w4015 _]
                    tunnel: w3991 -> [w4014 _]
                    tunnel: "Force Yank" -> [w4012 _]
                    tunnel: w3989 -> [w4011 w4201]
                    tunnel: [w4010 w4201] -> w3988
                    frame False {
                      n2604 = Negate(x=w4014) -> (-x=w4006:dbl)
                      n2605 = local write "Fl. High"(TRUE ("Fl. High")) -> ()
                      n2606 = Less?(x=w4015, y=w4006) -> (x < y?=w4013:bool)
                      n2607 = Or(x=w4012, y=w4013) -> (x .or. y?=w4008:bool)
                      n2608 = case shown="True" w4008 {
                        tunnel: w4011 -> [w4016 w4026]
                        tunnel: [w4016 w4025] -> w4010
                        tunnel: w4007 -> [_ w4024]
                        frame False {
                        }
                        frame True {
                          n2609 = flat-sequence {
                            tunnel: w4026 -> [w4032]
                            tunnel: w4024 -> [w4029]
                            tunnel: [w4031] -> w4023
                            tunnel: [w4030] -> w4022
                            tunnel: [w4029] -> w4021
                            tunnel: w4020 -> [w4028]
                            tunnel: [w4028] -> w4019
                            tunnel: w4018 -> [w4027]
                            tunnel: [w4027] -> w4017
                            tunnel: [w4103] -> w4025
                            tunnel: w4023 -> [w4103]
                            tunnel: w4022 -> [w4102]
                            tunnel: w4021 -> [w4101]
                            tunnel: w4019 -> [w4100]
                            tunnel: w4017 -> [w4099]
                            frame #0 {
                              n2610 = call <vilib>:"Beep.vi"() -> ()  [unwired: 12 in]
                              n2611 = local write "Waiting"(FALSE ("Waiting")) -> ()
                              n2612 = Increment(x=w4032) -> (x+1=w4031:i32)
                              n2613 = case shown="\"Image\"" w4029 {
                                tunnel: w4031 -> [_ w4037 _]
                                frame "Alarm", Default {
                                }
                                frame "Yank" {
                                n2614 = flat-sequence {
                                tunnel: w4037 -> [w4040]
                                tunnel: [w4039] -> w4036
                                tunnel: [w4038] -> w4035
                                tunnel: w4036 -> [w4050]
                                tunnel: w4035 -> [w4051]
                                frame #0 {
                                n2615 = local read "Yank Delay (s)"() -> (w4043:dbl)
                                n2616 = local read "N Array El"() -> (w4038:u8)
                                n2617 = Quotient & Remainder(x=w4040, y=w4038) -> (x-y*floor(x/y)=w4039:i32)  [unwired: 1 out]
